vi "TCP_Main.vi"() -> ()   [LabVIEW 2024]
uses:
  <vilib>/Platform/TimedLoop/XDataNode/timing_clust.ctl
  <vilib>/Platform/TimedLoop/XDataNode/nitl_modes.ctl
  <vilib>/Platform/TimedLoop/XDataNode/wakeup.ctl
  <vilib>/addons/Maxon Motor/EPOS2 CANopen/CANopen/sbCANopenBaseClass.lvclass
  <vilib>/platform/TimedLoop/XDataNode/XDataNode.xnode
  <vilib>/Platform/TimedLoop/XDataNode/XDNodeRunTimeDep.lvlib
panel:
  out "TCP Write Error":errorcluster
  out "TCP Read Error":errorcluster
  out "goal_Tensions":dbl[](array[numeric])
  out "ResetPID":bool
  in  "Motor_index":i32[](array[numeric])=[3, 6, 9, 12, 2, 7, 8, 13, 4, 5, 10, 11, 1, 14]
  out "canERROR":errorcluster[][](array[cluster])
  in  "Control Mode":string="O"
  in  "TARE":bool
  out "curr_Tensions":dbl[](array[numeric])
  out "DAQ Error":errorcluster
  out "Write Late?":bool
  out "Write Time [us]":i64
  in  "Tare_Tensions":dbl[](array[numeric])=[1.6875269817998764, 0.7228096971601798, 1.962272927280566, 2.6696462364433735, 2.7003690389898463, 3.088938448864716, 1.6430905755314908, 3.0754139877790347, 3.5546581214666455, 3.2737863413382597, 4.727265898547672, 2.6001067118162604, 1.980007529135911, 1.8614502099489874]
  in  "STOP CONTROLLER":bool
  # "TCP Read \"Error\" codes:\n\n66 - Client Disconnected\n56 - TCP Read time out (every 1ms if no msg comes in)\n0 - packet received"
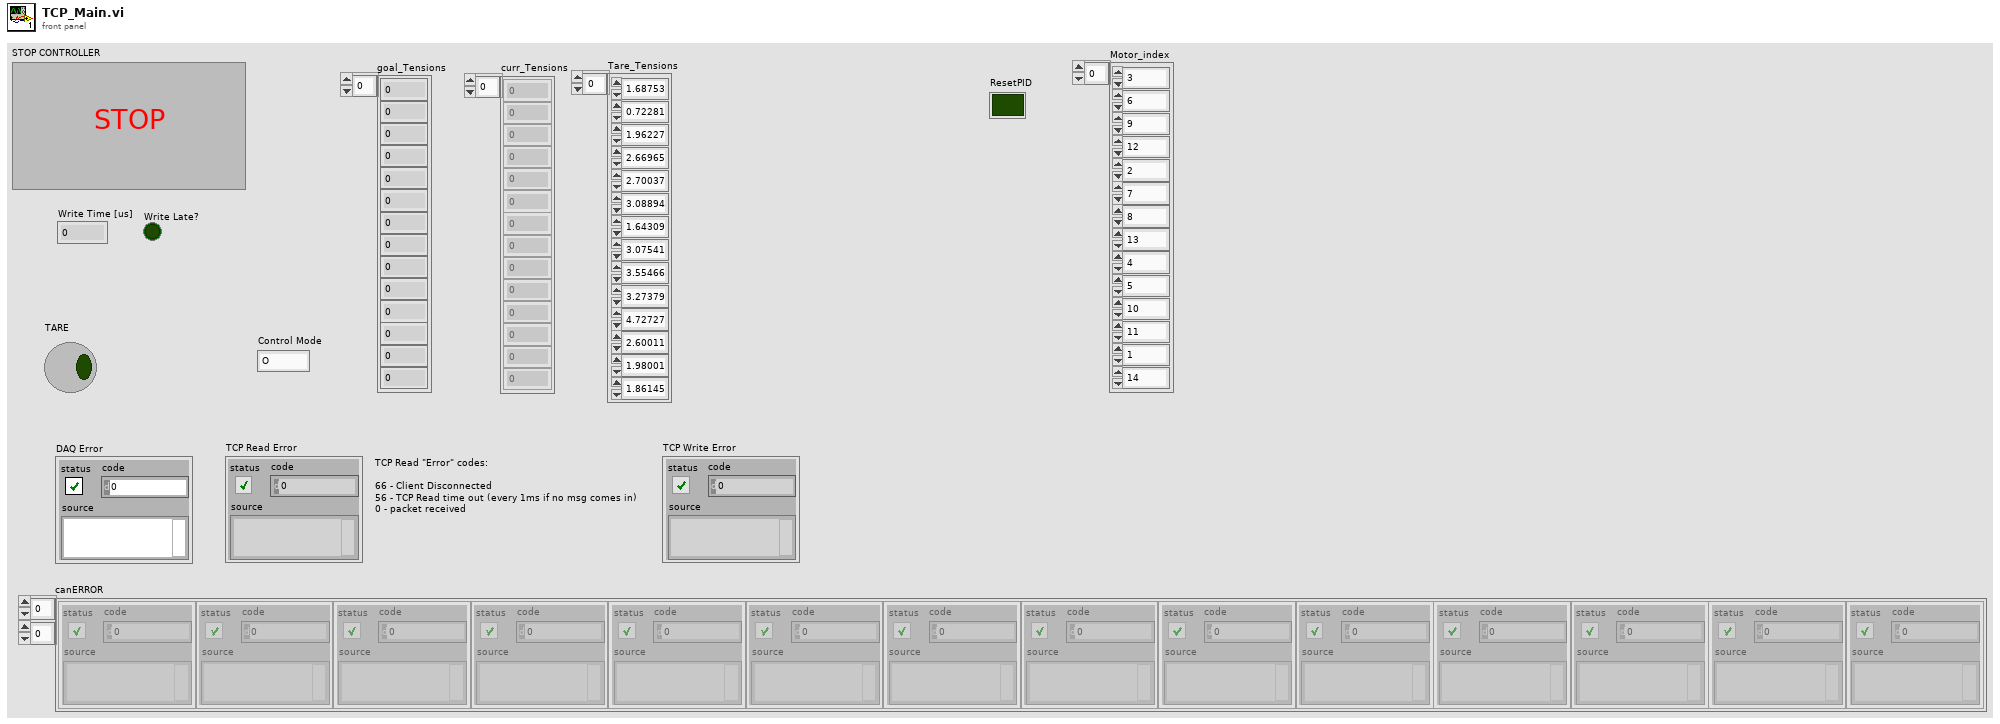
[diagram p1: front panel]
types:
  T1 = enum16{"Standard", "Buffered", "CRLF", "Immediate"}
  T2 = typedef "XDNodeRunTimeDep.lvlib/timing_clust.ctl" = cluster{"Expected End [f-1]":u64, "Actual End [f-1]":u64, "Finished Late? [f-1]":bool, "Expected End [i-1]":u64, "Actual End [i-1]":u64, "Finished Late? [i-1]":bool, "Expected Start [i]":u64, "Actual Start [i]":u64, "Expected Start [f]":u64, "Actual Start [f]":u64, "Source Name":string, "Structure Name":string, "Period":i64, "Deadline":i64, "Offset":i64, "Start":i64, "Priority":i32, "Timeout":i32, "Mode":T3, "Wakeup Reason":T4, "Error":errorcluster, "Source Type":string, "Secondary Source Type":string, "Global End Time":u64, "Global Start Time":u64, "Frame Duration":u64, "Iteration Duration":u64, "Assigned CPU":i32, "I/O Scan Engine Mode":u32}
  T3 = typedef "XDNodeRunTimeDep.lvlib/nitl_modes.ctl" = enum32{"No Change", "Process missed periods, maintain original phase", "Discard missed periods, maintain original phase", "Process missed periods, ignore original phase", "Discard missed periods, ignore original phase"}
  T4 = typedef "XDNodeRunTimeDep.lvlib/wakeup.ctl" = enum32{"Normal", "Aborted", "Asynchronous wakeup", "Timing source error", "Timed loop error", "Timeout"}
  T5 = cluster{"Array of Double":dbl[], "Array of Double":dbl[]}
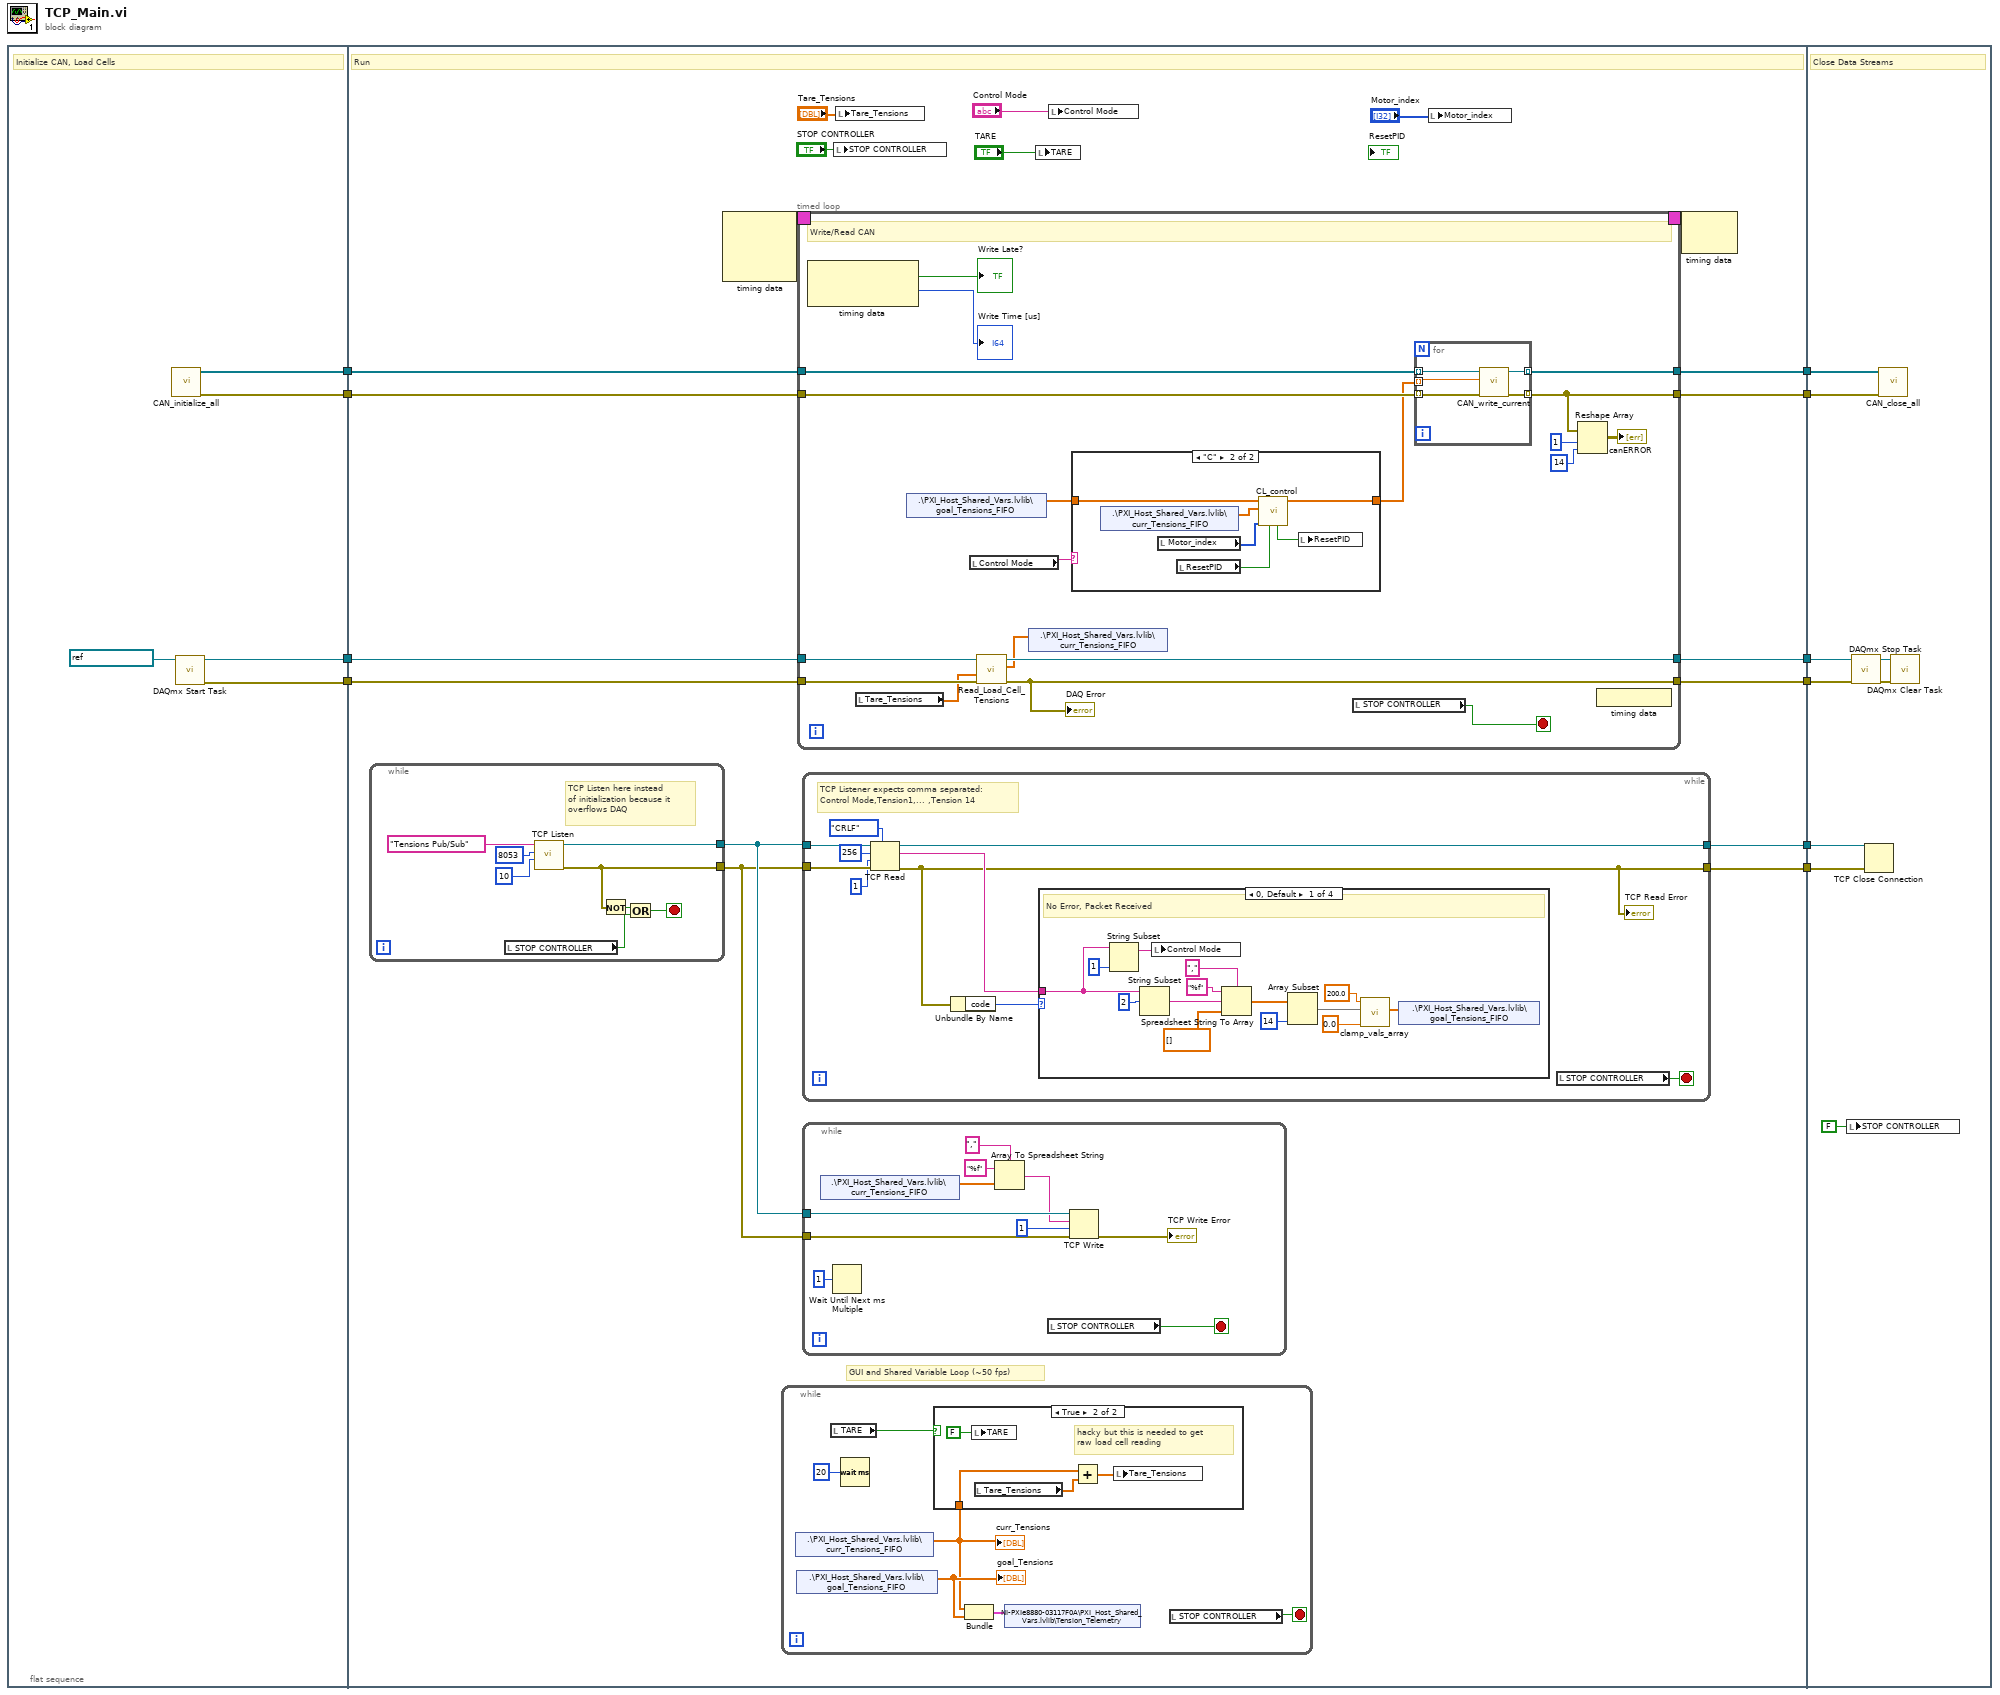
[diagram p0: block diagram]
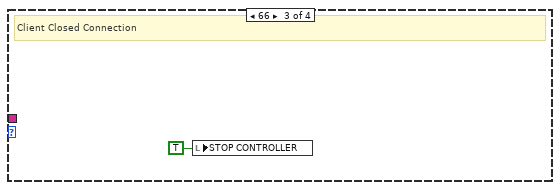
[diagram p3: hidden frame]
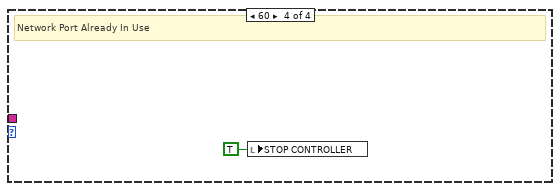
[diagram p4: hidden frame]
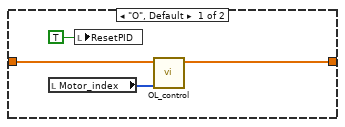
[diagram p6: hidden frame]
diagram:
  n1 = flat-sequence {
    tunnel: [w14] -> w10
    tunnel: [w15] -> w9
    tunnel: [w11] -> w6
    tunnel: [w12] -> w5
    tunnel: w10 -> [w32]
    tunnel: w9 -> [w31]
    tunnel: [w30] -> w8
    tunnel: [w29] -> w7
    tunnel: w6 -> [w27]
    tunnel: w5 -> [w26]
    tunnel: [w25] -> w4
    tunnel: [w24] -> w3
    tunnel: [w18] -> w2
    tunnel: [w19] -> w1
    tunnel: w8 -> [w137]
    tunnel: w7 -> [w136]
    tunnel: w4 -> [w133]
    tunnel: w3 -> [w132]
    tunnel: w2 -> [w130]
    tunnel: w1 -> [w129]
    frame #0 {
      # "Initialize CAN, Load Cells"
      n2 = call "CAN_initialize_all.vi"() -> ("Array of Canopen Sessions"=w15:refnum<class "sbCANopenBaseClass.lvclass">[], "Array of Error out's"=w14:errorcluster[])  [unwired: 5 in]
      n3 = call <vilib>:"DAQmx Start Task.vi"("task/channels in"=refnum<k21> "SCI_TenSen") -> ("task out"=w11:refnum<k21>, "error out"=w12:errorcluster)  [unwired: 13 in]
    }
    frame #1 {
      # "GUI and Shared Variable Loop (~50 fps)"
      # "Run"
      n4 = while {
        tunnel: [w45] -> w16
        tunnel: [w52] -> w17
        stop <- w47 stop-if-true
        # "TCP Listen here instead\nof initialization because it\noverflows DAQ"
        n5 = local read "STOP CONTROLLER"() -> (w48:bool)
        n6 = call <vilib>:"TCP Listen.vi"("timeout ms (wait forever: -1)"=10, "port"=u16 8053, "service name"="Tensions Pub/Sub") -> ("error out"=w45:errorcluster, "connection ID"=w52:refnum<k5>)  [unwired: 4 in, 3 out]
        n7 = Not(x=w45) -> (.not. x?=w46:bool)
        n8 = Or(x=w46, y=w48) -> (x .or. y?=w47:bool)
      }
      n9 = node-c288() -> (w34:T2)  [unwired: 3 in]
      n10 = while {
        stop <- w84 stop-if-true
        n11 = shared-variable ".\\PXI_Host_Shared_Vars.lvlib\\curr_Tensions_FIFO"() -> (w79:dbl[])  [unwired: 1 in, 1 out]
        "curr_Tensions" <- w79
        n12 = shared-variable ".\\PXI_Host_Shared_Vars.lvlib\\goal_Tensions_FIFO"() -> (w80:dbl[])  [unwired: 1 in, 1 out]
        "goal_Tensions" <- w80
        n13 = local read "TARE"() -> (w83:bool)
        n14 = Wait (ms)(milliseconds to wait=u32 20) -> ()  [unwired: 1 out]
        n15 = case shown="True" w83 {
          tunnel: w79 -> [_ w85]
          frame False {
          }
          frame True {
            # "hacky but this is needed to get \nraw load cell reading"
            n16 = local write "TARE"(FALSE ("TARE")) -> ()
            n17 = local read "Tare_Tensions"() -> (w87:dbl[])
            n18 = Add(x=w85, y=w87) -> (x+y=w88:dbl[])
            n19 = local write "Tare_Tensions"(w88) -> ()
          }
        }
        n20 = Bundle("Array of Double"=w79, "Array of Double"=w80) -> (w82:T5)  [unwired: 1 in]
        n21 = shared-variable "NI-PXIe8880-03117F0A\\PXI_Host_Shared_Vars.lvlib\\Tension_Telemetry"(w82) -> ()  [unwired: 1 in, 1 out]
        n22 = local read "STOP CONTROLLER"() -> (w84:bool)
      }
      n23 = timed-loop {
        tunnel: w32 -> [w99]
        tunnel: [w92] -> w30
        timing: w34 -> [_]
        timing-out: [_] -> w33
        tunnel: w31 -> [w100]
        tunnel: [w104] -> w29
        tunnel: w27 -> [w103]
        tunnel: w26 -> [w102]
        tunnel: [w101] -> w25
        tunnel: [w98] -> w24
        stop <- w105 stop-if-true
        # "Write/Read CAN"
        n24 = node-c288() -> (→"Write Late?":bool, →"Write Time [us]":i64)  [unwired: 1 in]
        n25 = local read "Tare_Tensions"() -> (w97:dbl[])
        n26 = shared-variable ".\\PXI_Host_Shared_Vars.lvlib\\goal_Tensions_FIFO"() -> (w89:dbl[])  [unwired: 1 in, 1 out]
        n27 = local read "Control Mode"() -> (w96:string)
        n28 = call "Read_Load_Cell_Tensions.vi"("error in (no error)"=w102, "Tare Tension"=w97, "Refnum in"=w103) -> ("error out"=w98:errorcluster, "Measured Cable Tensions"=w90:dbl[], "Refnum out"=w101:refnum<k21>)  [unwired: 4 in]
        "DAQ Error" <- w98
        n29 = shared-variable ".\\PXI_Host_Shared_Vars.lvlib\\curr_Tensions_FIFO"(w90) -> ()  [unwired: 1 in, 1 out]
        n30 = case shown="\"C\"" w96 {
          tunnel: [w111 w117] -> w95
          tunnel: w89 -> [w108 w112]
          frame "O", Default {
            n31 = local read "Motor_index"() -> (w110:i32[])
            n32 = local write "ResetPID"(TRUE) -> ()
            n33 = call "OL_control.vi"("Motor_index"=w110, "goal_Tensions"=w108) -> ("can_Current"=w111:dbl[])  [unwired: 9 in]
          }
          frame "C" {
            n34 = shared-variable ".\\PXI_Host_Shared_Vars.lvlib\\curr_Tensions_FIFO"() -> (w113:dbl[])  [unwired: 1 in, 1 out]
            n35 = local read "Motor_index"() -> (w116:i32[])
            n36 = local read "ResetPID"() -> (w115:bool)
            n37 = call "CL_control.vi"("ResetPID"=w115, "Motor_index"=w116, "curr_Tensions"=w113, "goal_Tensions"=w112) -> ("can_Current"=w117:dbl[], "Reset PID (output)"=w114:bool)  [unwired: 6 in]
            n38 = local write "ResetPID"(w114) -> ()
          }
        }
        n39 = local read "STOP CONTROLLER"() -> (w105:bool)
        n40 = for {
          tunnel: [w119] -> w104 mode=indexing
          tunnel: [w120] -> w92 mode=indexing
          tunnel: w100 -> [w122] mode=indexing
          tunnel: w99 -> [w121] mode=indexing
          tunnel: w95 -> [w118] mode=indexing
          n41 = call "CAN_write_current.vi"("error in"=w121, "Current Command [mA]"=w118, "CANopen Session In"=w122) -> ("error out"=w120:errorcluster, "CANopen Session Out"=w119:refnum<class "sbCANopenBaseClass.lvclass">)  [unwired: 7 in]
        }
        n42 = Reshape Array(w92, 1 ("dimension size"), 14 ("dimension size")) -> (→"canERROR":errorcluster[][])
        n43 = node-c288() -> ()  [unwired: 1 out]
      }
      n44 = while {
        tunnel: [w54] -> w18
        tunnel: [w62] -> w19
        tunnel: w16 -> [w60]
        tunnel: w17 -> [w59]
        stop <- w56 stop-if-true
        # "TCP Listener expects comma separated:\nControl Mode,Tension1,... ,Tension 14"
        n45 = TCP Read(connection ID=w59, bytes to read=256, error in (no error)=w60, 7:T1."CRLF" ("mode (standard)"), 9:1 ("timeout ms (25000)")) -> (connection ID out=w62:refnum<k5>, data out=w61:string, error out=w54:errorcluster)
        "TCP Read Error" <- w54
        n46 = Unbundle By Name(w54) -> ("code"=w55:i32)
        n47 = case shown="0, Default" w55 {
          tunnel: w61 -> [w74 _ _ _]
          frame 0, Default {
            # "No Error, Packet Received"
            n48 = String Subset(string=w74, length (rest)=1 ("length (rest)")) -> (substring=w75:string)  [unwired: 1 in]
            n49 = String Subset(string=w74, offset (0)=2) -> (substring=w72:string)  [unwired: 1 in]
            n50 = local write "Control Mode"(w75) -> ()
            n51 = Spreadsheet String To Array(delimiter (Tab)=",", format string="%f", spreadsheet string=w72, array type (2D Dbl)=dbl[] []) -> (array=w67:dbl[])
            n52 = Array Subset(array=w67, length=14) -> (w64:dbl[])  [unwired: 1 in]
            n53 = call "clamp_vals_array.vi"("Min Val"=0.0, "Input Array"=w64, "Max Val"=200.0) -> ("Output Array"=w63:dbl[])  [unwired: 8 in]
            n54 = shared-variable ".\\PXI_Host_Shared_Vars.lvlib\\goal_Tensions_FIFO"(w63) -> ()  [unwired: 1 in, 1 out]
          }
          frame 56 {
            # "continue"
            # "Time out Error"
          }
          frame 66 {
            # "Client Closed Connection"
            n55 = local write "STOP CONTROLLER"(TRUE ("STOP CONTROLLER")) -> ()
          }
          frame 60 {
            # "Network Port Already In Use"
            n56 = local write "STOP CONTROLLER"(TRUE ("STOP CONTROLLER")) -> ()
          }
        }
        n57 = local read "STOP CONTROLLER"() -> (w56:bool)
      }
      n58 = while {
        tunnel: w17 -> [w43]
        tunnel: w16 -> [w42]
        stop <- w44 stop-if-true
        n59 = shared-variable ".\\PXI_Host_Shared_Vars.lvlib\\curr_Tensions_FIFO"() -> (w40:dbl[])  [unwired: 1 in, 1 out]
        n60 = Wait Until Next ms Multiple(millisecond multiple=u32 1) -> ()  [unwired: 1 out]
        n61 = Array To Spreadsheet String(delimiter (Tab)=",", array=w40, 3:"%f" ("format string")) -> (spreadsheet string=w37:string)
        n62 = local read "STOP CONTROLLER"() -> (w44:bool)
        n63 = TCP Write(connection ID=w43, data in=w37, error in (no error)=w42, 9:1 ("timeout ms (25000)")) -> (error out=→"TCP Write Error":errorcluster)  [unwired: 2 out]
      }
      n64 = local write "STOP CONTROLLER"("STOP CONTROLLER") -> ()
      n65 = local write "Tare_Tensions"("Tare_Tensions") -> ()
      n66 = local write "TARE"("TARE") -> ()
      n67 = local write "Control Mode"("Control Mode") -> ()
      n68 = local write "Motor_index"("Motor_index") -> ()
      n69 = node-c288(w33) -> ()  [unwired: 1 out]
    }
    frame #2 {
      # "Close Data Streams"
      n70 = local write "STOP CONTROLLER"(FALSE ("STOP CONTROLLER")) -> ()
      n71 = call <vilib>:"DAQmx Stop Task.vi"("task/channels in"=w133, "error in"=w132) -> ("task out"=w134:refnum<k21>, "error out"=w135:errorcluster)  [unwired: 12 in]
      n72 = TCP Close Connection(connection ID=w129, error in (no error)=w130) -> ()  [unwired: 1 in, 2 out]
      n73 = call "CAN_close_all.vi"("Input Error out array"=w137, "Input CANopen Sessions array"=w136) -> ()  [unwired: 10 in]
      n74 = call <vilib>:"DAQmx Clear Task.vi"("task in"=w134, "error in"=w135) -> ()  [unwired: 13 in, 1 out]
    }
  }
